vi "Init RGB Color.vi"(0 "RGB Color in":refnum<class "RGB Color.lvclass">, 5 "R (0)":u8, 7 "G (0)":u8, 9 "B (0)":u8, 11 "error in (no error)":errorcluster) -> (4 "RGB Color out":refnum<class "RGB Color.lvclass">, 15 "error out":errorcluster)   [LabVIEW 2020, in "RGB Color.lvclass"]
doc: "Initialize an RGB color"
uses:
  RGB Color.lvclass
  RGB Color.lvclass/RGB Color.ctl
panel:
  # "expressionflow.com"
  # "Copyright (c) 2008 Tomi Maila. All rights reserved."
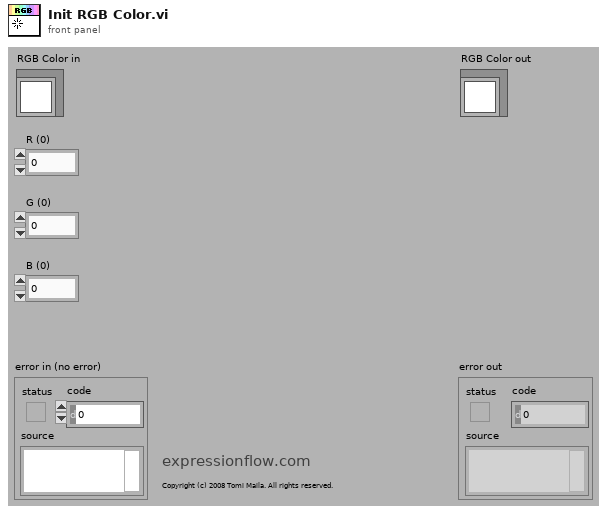
[diagram p1: front panel]
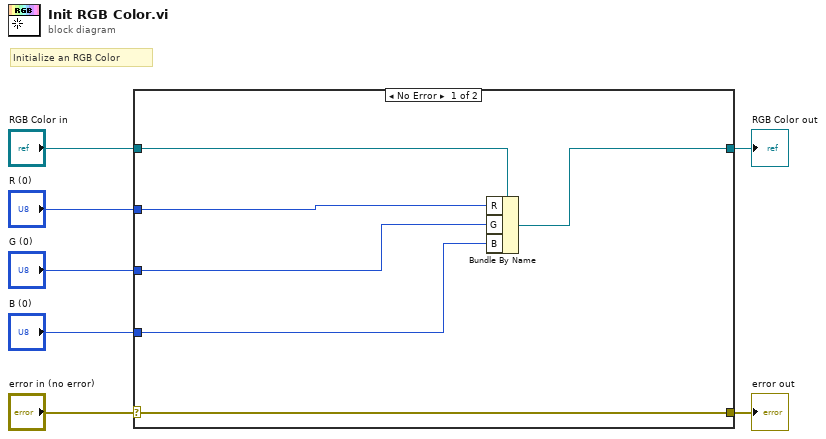
[diagram p0: block diagram]
diagram:
  # "Initialize an RGB Color"
  n1 = case shown="No Error" "error in (no error)" {
    selector: "error in (no error)" -> [w13 w15]
    tunnel: [w13 w15] -> w6
    tunnel: [w11 w14] -> w4
    tunnel: "RGB Color in" -> [w12 w14]
    tunnel: "R (0)" -> [w10 _]
    tunnel: "G (0)" -> [w9 _]
    tunnel: "B (0)" -> [w8 _]
    frame No Error {
      n2 = Bundle By Name(cluster=w12, "R"=w10, "G"=w9, "B"=w8) -> (w11:refnum<class "RGB Color.lvclass">)
    }
    frame Error {
    }
  }
  "error out" <- w6
  "RGB Color out" <- w4
